vi "ParseVariable.vi"(8 "error in":errorcluster, 11 "Variant":variant) -> (0 "error out":errorcluster, 2 "Parameter":string, 3 "MapName":string)   [LabVIEW 2016, in "SeqProcessor.lvlib"]
uses:
  SeqProcessor.lvlib
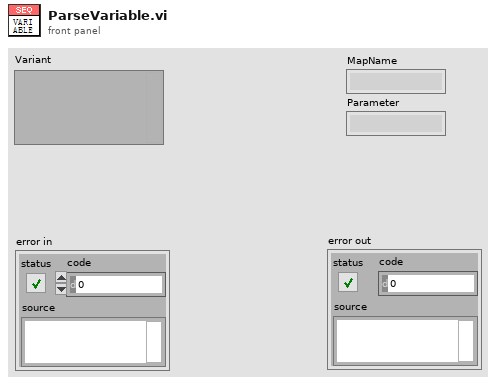
[diagram p1: front panel]
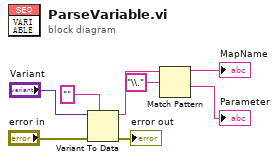
[diagram p0: block diagram]
diagram:
  n1 = Variant To Data(error in="error in", type="" ("regular expression"), Variant="Variant") -> (data=w6:string, error out=→"error out":errorcluster)
  n2 = Match Pattern(string=w6, regular expression="\\.") -> (before substring=→"MapName":string, after substring=→"Parameter":string)  [unwired: 1 in, 2 out]
